vi "FW_Read.vi"(8 "error in (no error)":errorcluster, 10 "Write buffer":string, 11 "VISA Refnum in":refnum<visa-resource-name>) -> (0 "error out":errorcluster, 2 "FW_Version":u32, 3 "read buffer":string)   [LabVIEW 2018]
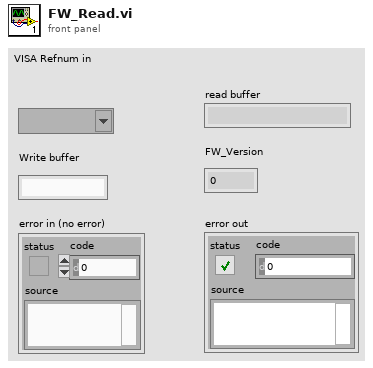
[diagram p1: front panel]
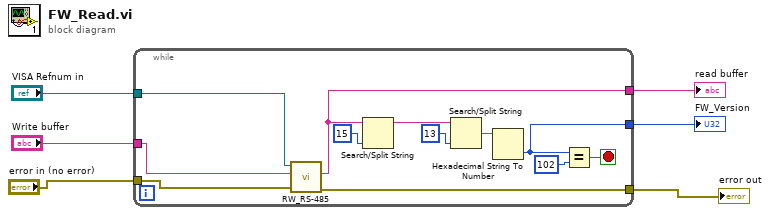
[diagram p0: block diagram]
diagram:
  n1 = while {
    tunnel: [w12] -> w1
    tunnel: [w11] -> w2
    tunnel: "VISA Refnum in" -> [w10]
    tunnel: "error in (no error)" -> [w9]
    tunnel: [w8] -> w5
    tunnel: "Write buffer" -> [w7]
    stop <- w13 stop-if-true
    n2 = call "RW_RS-485.vi"("error in (no error)"=w9, "Initial Command"=w7, "VISA Refnum in"=w10) -> ("error out"=w8:errorcluster, "read buffer"=w11:string)  [unwired: 7 in]
    n3 = Search/Split String(string=w11, offset (0)=15) -> (substring before match=w16:string)  [unwired: 1 in, 2 out]
    n4 = Search/Split String(string=w16, offset (0)=13) -> (match + rest of string=w15:string)  [unwired: 1 in, 2 out]
    n5 = Hexadecimal String To Number(string=w15) -> (number=w12:u32)  [unwired: 2 in, 1 out]
    n6 = Equal?(x=w12, y=u32 102) -> (x = y?=w13:bool)
  }
  "FW_Version" <- w1
  "read buffer" <- w2
  "error out" <- w5
